vi "IB_ReadLog (Outside).vi"() -> (6 "Array":dbl[](array[numeric]))   [LabVIEW 2013]
panel:
  out "F":cluster{timestamp[], dbl[]}(graph)
  out "E":cluster{timestamp[], dbl[]}(graph)
  out "D":cluster{timestamp[], dbl[]}(graph)
  out "C":cluster{timestamp[], dbl[]}(graph)
  out "Time Stamp":timestamp[](array[timestamp])
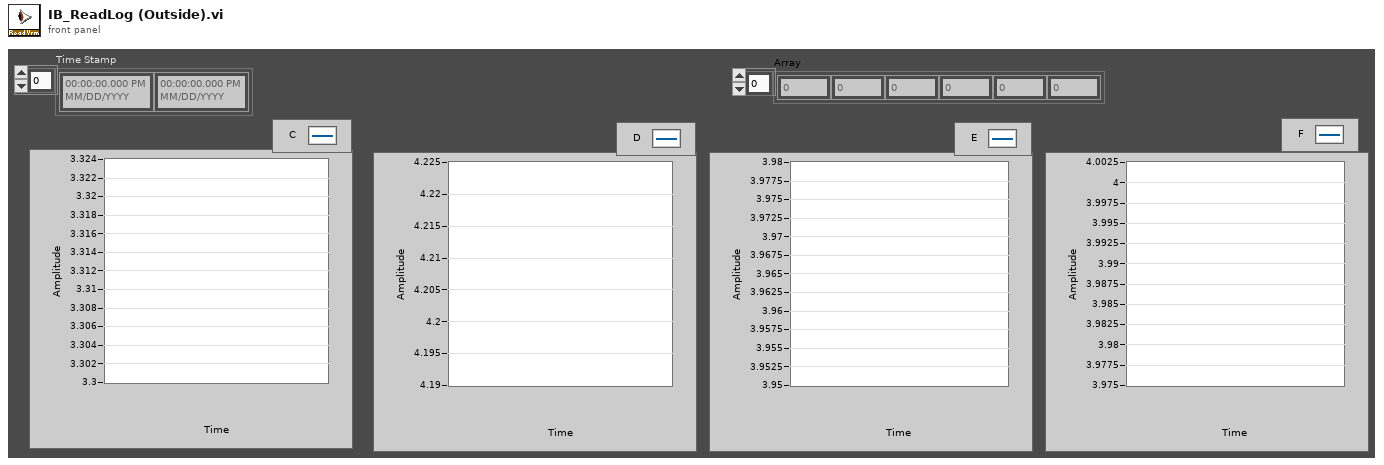
[diagram p1: front panel]
types:
  T1 = cluster{"second":i32, "minute":i32, "hour":i32, "day of month":i32, "month":i32, "year":i32, "day of week":i32, "day of year":i32, "is DST":i32}
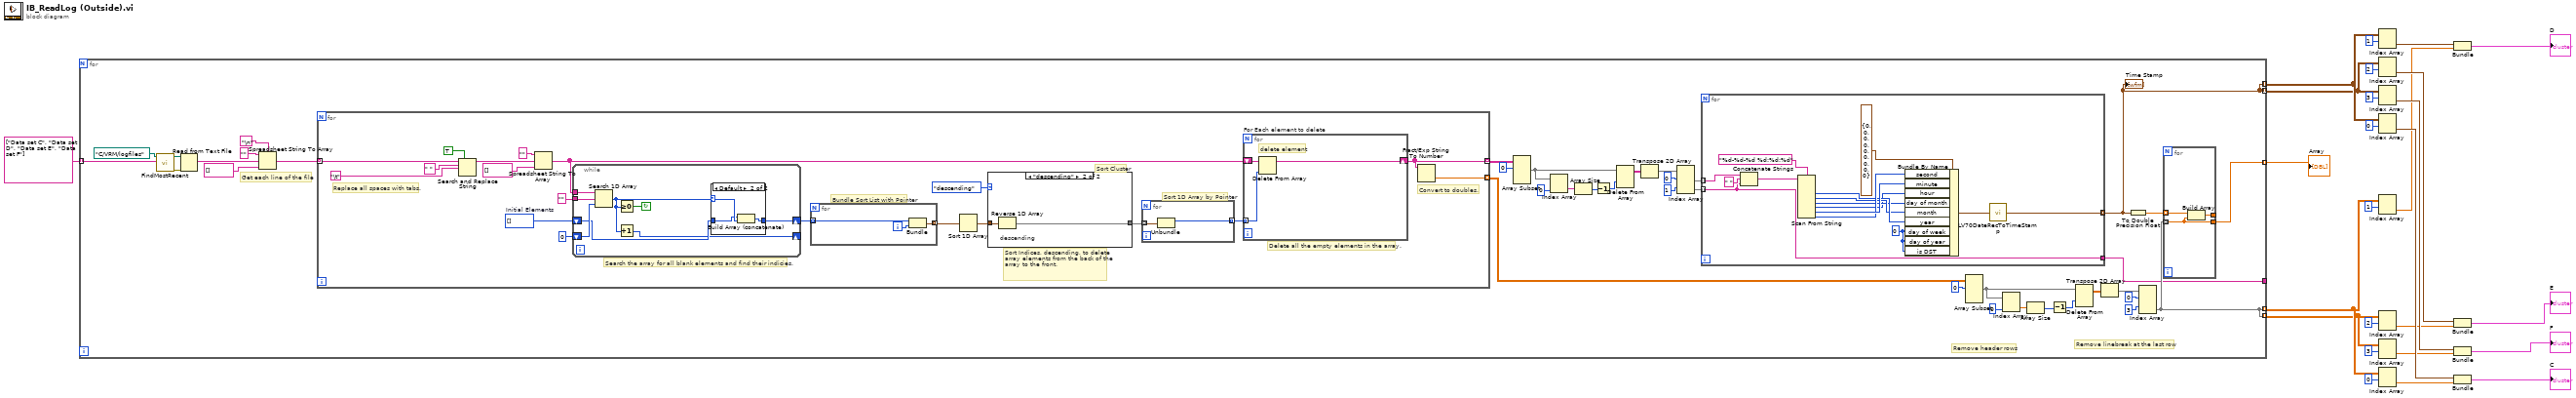
[diagram p0: block diagram]
diagram:
  n1 = for {
    tunnel: string[] ["Data set C", "Data set D", "Data set E", "Data set F"] -> [w31] mode=indexing
    tunnel: [w30] -> w19 mode=indexing
    tunnel: [w29] -> w18 mode=indexing
    tunnel: [w30] -> w13 mode=indexing
    tunnel: [w29] -> w12 mode=indexing
    tunnel: [w28] -> _
    tunnel: [w27] -> w1 mode=indexing
    # "Remove linebreak at the last row"
    # "Remove header rows"
    # "Get each line of the file"
    n2 = call "FindMostRecent.vi"("Filename Pattern"=w31, "Folder Path In"=path "C:/VRM/logfiles") -> ("error out"=w32:errorcluster, "File Path for the Newest File"=w33:path)  [unwired: 8 in]
    n3 = Read from Text File(file (use dialog)=w33, error in=w32) -> (text=w64:string)  [unwired: 5 out]
    n4 = Spreadsheet String To Array(delimiter (Tab)="\n", format string="", spreadsheet string=w64, array type (2D Dbl)=string[] []) -> (array=w60:string[])
    n5 = for {
      tunnel: w60 -> [w101] mode=indexing
      tunnel: [w83] -> w42 mode=indexing
      tunnel: [w84] -> w56 mode=indexing
      w93 = i32[] []  # Initial Elements
      # "Convert to doubles."
      # "Delete all the empty elements in the array."
      # "Search the array for all blank elements and find their indicies."
      # "Replace all spaces with tabs."
      # "Sort 1D Array by Pointer"
      # "Sort Cluster"
      # "Bundle Sort List with Pointer"
      # "Sort Indices, descending, to delete array elements from the back of the array to the front."
      n6 = Search and Replace String(replace all?=TRUE ("replace all? (F)"), input string=w101, search string=" ", replace string="\t") -> (result string=w96:string)  [unwired: 1 in, 6 out]
      n7 = Spreadsheet String To Array(format string="", spreadsheet string=w96, array type (2D Dbl)=string[] []) -> (array=w91:string[])  [unwired: 1 out]
      n8 = while {
        shift-right: [w113] -> _
        shift-left: 0 -> [w120]
        shift-right: [w117] -> w87
        shift-left: w93 -> [w118]
        tunnel: w91 -> [w119]
        tunnel: "" ("Element Data") -> [w116]
        stop <- w114 continue-if-true
        n9 = Search 1D Array(1D array=w119, element=w116, start index (0)=w120) -> (index of element=w115:i32)
        n10 = Greater Or Equal To 0?(x=w115) -> (x >= 0?=w114:bool)
        n11 = Increment(x=w115) -> (x+1=w113:i32)
        n12 = case shown="Default" w115 {
          selector: w115 -> [_ w124]
          tunnel: w118 -> [w121 w123]
          tunnel: [w121 w122] -> w117
          frame -1 {
          }
          frame Default {
            n13 = Build Array (concatenate)(w123, w124) -> (w122:i32[])
          }
        }
      }
      n14 = for {
        tunnel: w87 -> [w104] mode=indexing
        tunnel: [w102] -> w89 mode=indexing
        i -> [w103]
        n15 = Bundle("index of element"=w104, w103) -> (w102:cluster{"index of element":i32, i32})  [unwired: 1 out]
      }
      n16 = Sort 1D Array(array=w89) -> (sorted array=w88:cluster{"index of element":i32, i32}[])
      n17 = case shown="\"descending\"" enum16{"ascending", "descending"}."descending" ("Order") {
        tunnel: [w105 w106] -> w90
        tunnel: w88 -> [w105 w107]
        frame "ascending", Default {
        }
        frame "descending" {
          # "descending"
          n18 = Reverse 1D Array(array=w107) -> (reversed array=w106:cluster{"index of element":i32, i32}[])
        }
      }
      n19 = for {
        tunnel: w90 -> [w109] mode=indexing
        tunnel: [w108] -> w85 mode=indexing
        n20 = Unbundle(w109) -> ("index of element"=w108:i32)  [unwired: 1 out]
      }
      n21 = for "For Each element to delete" {
        tunnel: w85 -> [w112] mode=indexing
        shift-right: [w111] -> w83
        shift-left: w91 -> [w110]
        # "delete element"
        n22 = Delete From Array(array=w110, index=w112) -> (array with subset deleted=w111:string[])  [unwired: 1 in, 1 out]
      }
      n23 = Fract/Exp String To Number(string=w83) -> (number=w84:dbl[])  [unwired: 4 out]
    }
    n24 = Array Subset(array=w42, index (row)=0 ("index")) -> (w43:string[][])  [unwired: 3 in]
    n25 = Index Array(array=w43, index (col)=0 ("disabled index (col)")) -> (element=w46:string[])  [unwired: 1 in]
    n26 = Array Size(array=w46) -> (size(s)=w45:i32)
    n27 = Decrement(x=w45) -> (x-1=w44:i32)
    n28 = Delete From Array(array=w43, index (row)=w44) -> (array with subset deleted=w41:string[][])  [unwired: 2 in, 1 out]
    n29 = Transpose 2D Array(2D array=w41) -> (transposed array=w38:string[][])
    n30 = Index Array(array=w38, index (row) #1=0 ("disabled index (col)"), index (row) #2=1 ("index (col)")) -> (element #1=w37:string[], element #2=w36:string[])  [unwired: 2 in]
    n31 = for {
      tunnel: w37 -> [w78] mode=indexing
      tunnel: w36 -> [w65] mode=indexing
      tunnel: [w66] -> w30 mode=indexing
      tunnel: [w65] -> w28
      w75 = 0
      n32 = Concatenate Strings(w78, " " ("string"), w65) -> (w67:string)
      n33 = Scan From String "Scan From String"(format string="%d-%d-%d %d:%d:%d", input string=w67) -> (output 1=w72:i32, output 2=w71:i32, output 3=w70:i32, output 4=w69:i32, output 5=w74:i32, output 6=w73:i32)  [unwired: 8 in, 3 out]
      n34 = Bundle By Name(cluster=T1 {"second"=0, "minute"=0, "hour"=0, "day of month"=0, "month"=0, "year"=0, "day of week"=0, "day of year"=0, "is DST"=0} ("date time rec"), "second"=w73, "minute"=w74, "hour"=w69, "day of month"=w70, "month"=w71, "year"=w72, "day of week"=w75, "day of year"=w75, "is DST"=w75) -> (w76:T1)
      n35 = call <vilib>:"LV70DateRecToTimeStamp.vi"("date time rec"=w76) -> ("Time Stamp"=w66:timestamp)
    }
    "Time Stamp" <- w30
    n36 = Array Subset(array=w56, index (row)=0 ("index")) -> (w50:dbl[][])  [unwired: 3 in]
    n37 = Index Array(array=w50, index (col)=0 ("disabled index (col)")) -> (element=w54:dbl[])  [unwired: 1 in]
    n38 = Array Size(array=w54) -> (size(s)=w52:i32)
    n39 = Decrement(x=w52) -> (x-1=w51:i32)
    n40 = Delete From Array(array=w50, index (row)=w51) -> (array with subset deleted=w53:dbl[][])  [unwired: 2 in, 1 out]
    n41 = Transpose 2D Array(2D array=w53) -> (transposed array=w49:dbl[][])
    n42 = To Double Precision Float(number=w30) -> (double precision float=w35:dbl[])
    n43 = Index Array(array=w49, index (row) #1=0 ("index (row)"), index (row) #2=3 ("index (row)")) -> (element #2=w29:dbl[])  [unwired: 2 in, 1 out]
    n44 = for {
      tunnel: w29 -> [w80] mode=indexing
      tunnel: [w82] -> _
      tunnel: w35 -> [w81] mode=indexing
      tunnel: [w80] -> w27
      n45 = Build Array(w81, w80) -> (w82:dbl[])
    }
  }
  "Array" <- w1
  n46 = Index Array(array=w18, index (row)=1) -> (element=w6:dbl[])  [unwired: 1 in]
  n47 = Index Array(array=w12, index (row)=2) -> (element=w8:dbl[])  [unwired: 1 in]
  n48 = Index Array(array=w12, index (row)=3) -> (element=w10:dbl[])  [unwired: 1 in]
  n49 = Index Array(array=w18, index (row)=0) -> (element=w22:dbl[])  [unwired: 1 in]
  n50 = Index Array(array=w19, index (row)=1) -> (element=w7:timestamp[])  [unwired: 1 in]
  n51 = Index Array(array=w13, index (row)=2) -> (element=w9:timestamp[])  [unwired: 1 in]
  n52 = Index Array(array=w13, index (row)=3) -> (element=w11:timestamp[])  [unwired: 1 in]
  n53 = Index Array(array=w19, index (row)=0) -> (element=w24:timestamp[])  [unwired: 1 in]
  n54 = Bundle(w7, w6) -> (→"D":cluster{timestamp[], dbl[]})  [unwired: 1 in]
  n55 = Bundle(w9, w8) -> (→"E":cluster{timestamp[], dbl[]})  [unwired: 1 in]
  n56 = Bundle(w11, w10) -> (→"F":cluster{timestamp[], dbl[]})  [unwired: 1 in]
  n57 = Bundle(w24, w22) -> (→"C":cluster{timestamp[], dbl[]})  [unwired: 1 in]
